vi "Set Basic FP Settings.vi"(8 "error in (no error)":errorcluster, 10 "basic fp settings":T1, 11 "vi reference":refnum<vi>) -> (0 "error out":errorcluster, 3 "vi reference out":refnum<vi>)   [LabVIEW 2020]
uses:
  Basic FP Settings--cluster.ctl
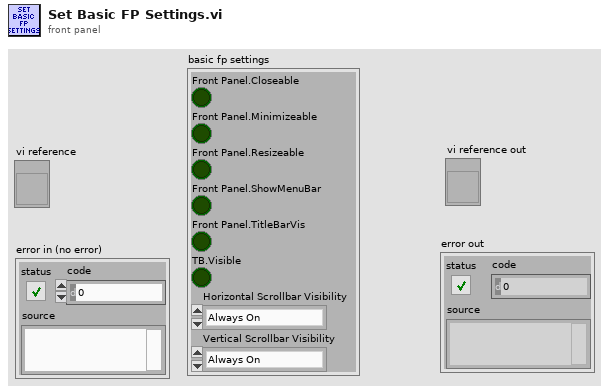
[diagram p1: front panel]
types:
  T1 = typedef "Basic FP Settings--cluster.ctl" = cluster{"Front Panel.Closeable":bool, "Front Panel.Minimizeable":bool, "Front Panel.Resizeable":bool, "Front Panel.ShowMenuBar":bool, "Front Panel.TitleBarVis":bool, "TB.Visible":bool, "Horizontal Scrollbar Visibility":enum16{"Always On", "Always Off", "Off While Running"}, "Vertical Scrollbar Visibility":enum16{"Always On", "Always Off", "Off While Running"}}
  T2 = enum16{"Always On", "Always Off", "Off While Running"}
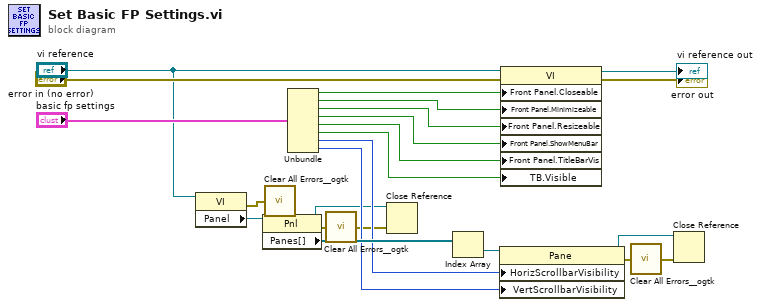
[diagram p0: block diagram]
diagram:
  n1 = property class="VI"(reference="vi reference") -> (error out=w7:errorcluster, "Panel"=w10:refnum<vi>)  [unwired: 1 in, 1 out]
  n2 = property class="Pnl"(reference=w10) -> (reference out=w3:refnum<vi>, error out=w6:errorcluster, "Panes[]"=w12:refnum<vi>[])  [unwired: 1 in]
  n3 = call <userlib>:"Clear All Errors__ogtk.vi"("Error In"=w7) -> ()  [unwired: 3 in, 1 out]
  n4 = Unbundle("basic fp settings") -> ("Front Panel.Closeable"=w22:bool, "Front Panel.Minimizeable"=w21:bool, "Front Panel.Resizeable"=w20:bool, "Front Panel.ShowMenuBar"=w19:bool, "Front Panel.TitleBarVis"=w18:bool, "TB.Visible"=w17:bool, "Horizontal Scrollbar Visibility"=w9:T2, "Vertical Scrollbar Visibility"=w8:T2)
  n5 = call <userlib>:"Clear All Errors__ogtk.vi"("Error In"=w6) -> ("Error Out"=w4:errorcluster)  [unwired: 3 in]
  n6 = Close Reference(reference=w3, error in (no error)=w4) -> ()  [unwired: 1 out]
  n7 = Index Array(array=w12) -> (element=w13:refnum<vi>)  [unwired: 1 in]
  n8 = property class="Pane"(reference=w13, "HorizScrollbarVisibility"=w9, "VertScrollbarVisibility"=w8) -> (reference out=w1:refnum<vi>, error out=w5:errorcluster)  [unwired: 1 in]
  n9 = property class="VI"(reference="vi reference", error in="error in (no error)", "Front Panel.Closeable"=w22, "Front Panel.Minimizeable"=w21, "Front Panel.Resizeable"=w20, "Front Panel.ShowMenuBar"=w19, "Front Panel.TitleBarVis"=w18, "TB.Visible"=w17) -> (reference out=→"vi reference out":refnum<vi>, error out=→"error out":errorcluster)
  n10 = call <userlib>:"Clear All Errors__ogtk.vi"("Error In"=w5) -> ("Error Out"=w2:errorcluster)  [unwired: 3 in]
  n11 = Close Reference(reference=w1, error in (no error)=w2) -> ()  [unwired: 1 out]
